vi "Write String.vi"(8 "error in (no error)":errorcluster, 11 "String":string) -> (0 "error out":errorcluster)   [LabVIEW 2015]
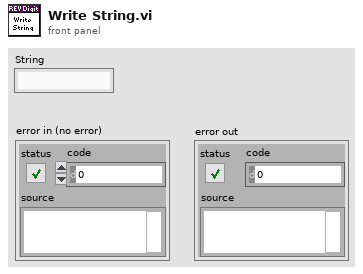
[diagram p1: front panel]
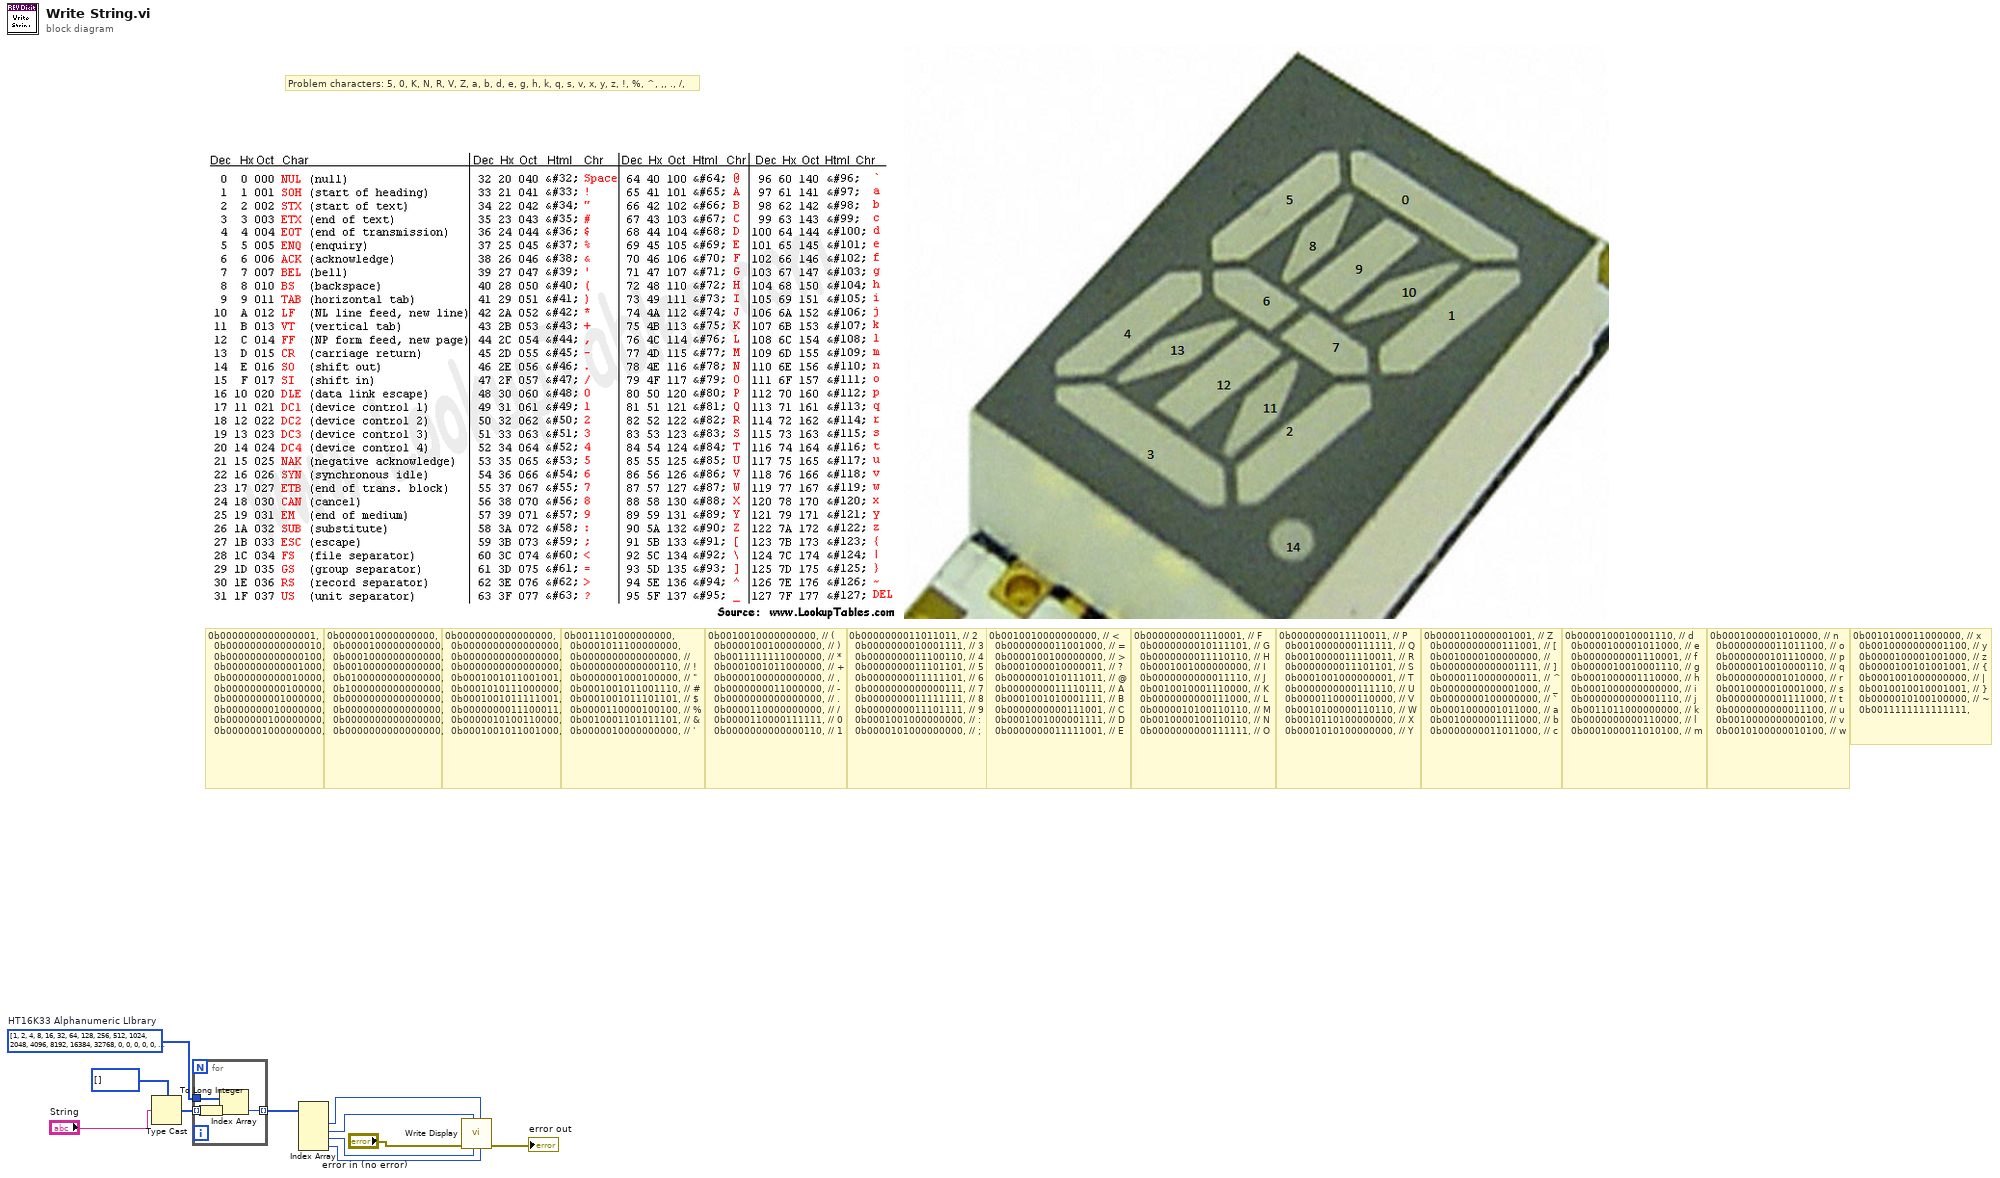
[diagram p0: block diagram]
diagram:
  w7 = u16[] [1, 2, 4, 8, 16, 32, 64, 128, 256, 512, 1024, 2048, 4096, 8192, 16384, 32768, 0, 0, 0, 0, 0, 0, 0, 0, 4809, 5568, 4857, 227, 1328, 4808, 14848, 5888, 0, 6, 544, 4814, 4845, 3108, 9053, 1024, 9216, 2304, 16320, 4800, 2048, 192, 0, 3072, 9279, 6, 219, 143, 230, 237, 253, 7, 255, 239, 4608, 2560, 9216, 200, 2304, 4227, 699, 247, 4751, 57, 4623, 249, 113, 189, 246, 4608, 30, 9328, 56, 1334, 8502, 63, 243, 8255, 8435, 237, 4609, 62, 3120, 10294, 11520, 5376, 3081, 57, 8448, 15, 3075, 8, 256, 4184, 8312, 216, 2190, 2136, 113, 1166, 4208, 4096, 14, 13824, 48, 4308, 4176, 220, 368, 1158, 80, 8328, 120, 28, 8196, 10260, 10432, 8204, 2120, 2377, 4608, 9353, 1312, 16383]  # HT16K33 Alphanumeric LIbrary
  # "Problem characters: 5, 0, K, N, R, V, Z, a, b, d, e, g, h, k, q, s, v, x, y, z, !, %, ^, ,, ., /,"
  # "0b0010100011000000, // x\n\t\t0b0010000000001100, // y\n\t\t0b0000100001001000, // z\n\t\t0b0000100101001001, // {\n\t\t0b0001001000000000, // |\n\t\t0b0010010010001001, // }\n\t\t0b0000010100100000, // ~\n\t\t0b0011111111111111,"
  # "0b0001000001010000, // n\n\t\t0b0000000011011100, // o\n\t\t0b0000000101110000, // p\n\t\t0b0000010010000110, // q\n\t\t0b0000000001010000, // r\n\t\t0b0010000010001000, // s\n\t\t0b0000000001111000, // t\n\t\t0b0000000000011100, // u\n\t\t0b0010000000000100, // v\n\t\t0b0010100000010100, // w"
  # "0b0000100010001110, // d\n\t\t0b0000100001011000, // e\n\t\t0b0000000001110001, // f\n\t\t0b0000010010001110, // g\n\t\t0b0001000001110000, // h\n\t\t0b0001000000000000, // i\n\t\t0b0000000000001110, // j\n\t\t0b0011011000000000, // k\n\t\t0b0000000000110000, // l\n\t\t0b0001000011010100, // m"
  # "0b0000000000000001,\n\t\t0b0000000000000010,\n\t\t0b0000000000000100,\n\t\t0b0000000000001000,\n\t\t0b0000000000010000,\n\t\t0b0000000000100000,\n\t\t0b0000000001000000,\n\t\t0b0000000010000000,\n\t\t0b0000000100000000,\n\t\t0b0000001000000000,"
  # "0b0000110000001001, // Z\n\t\t0b0000000000111001, // [\n\t\t0b0010000100000000, //\n\t\t0b0000000000001111, // ]\n\t\t0b0000110000000011, // ^\n\t\t0b0000000000001000, // _\n\t\t0b0000000100000000, // `\n\t\t0b0001000001011000, // a\n\t\t0b0010000001111000, // b\n\t\t0b0000000011011000, // c"
  # "0b0000000011110011, // P\n\t\t0b0010000000111111, // Q\n\t\t0b0010000011110011, // R\n\t\t0b0000000011101101, // S\n\t\t0b0001001000000001, // T\n\t\t0b0000000000111110, // U\n\t\t0b0000110000110000, // V\n\t\t0b0010100000110110, // W\n\t\t0b0010110100000000, // X\n\t\t0b0001010100000000, // Y"
  # "0b0000000001110001, // F\n\t\t0b0000000010111101, // G\n\t\t0b0000000011110110, // H\n\t\t0b0001001000000000, // I\n\t\t0b0000000000011110, // J\n\t\t0b0010010001110000, // K\n\t\t0b0000000000111000, // L\n\t\t0b0000010100110110, // M\n\t\t0b0010000100110110, // N\n\t\t0b0000000000111111, // O"
  # "0b0010010000000000, // <\n\t\t0b0000000011001000, // =\n\t\t0b0000100100000000, // >\n\t\t0b0001000010000011, // ?\n\t\t0b0000001010111011, // @\n\t\t0b0000000011110111, // A\n\t\t0b0001001010001111, // B\n\t\t0b0000000000111001, // C\n\t\t0b0001001000001111, // D\n\t\t0b0000000011111001, // E"
  # "0b0000000011011011, // 2\n\t\t0b0000000010001111, // 3\n\t\t0b0000000011100110, // 4\n\t\t0b0000000011101101, // 5\n\t\t0b0000000011111101, // 6\n\t\t0b0000000000000111, // 7\n\t\t0b0000000011111111, // 8\n\t\t0b0000000011101111, // 9\n\t\t0b0001001000000000, // :\n\t\t0b0000101000000000, // ;"
  # "0b0010010000000000, // (\n\t\t0b0000100100000000, // )\n\t\t0b0011111111000000, // *\n\t\t0b0001001011000000, // +\n\t\t0b0000100000000000, // ,\n\t\t0b0000000011000000, // -\n\t\t0b0000000000000000, // .\n\t\t0b0000110000000000, // /\n\t\t0b0000110000111111, // 0\n\t\t0b0000000000000110, // 1"
  # "0b0011101000000000,\n\t\t0b0001011100000000,\n\t\t0b0000000000000000, //\n\t\t0b0000000000000110, // !\n\t\t0b0000001000100000, // \"\n\t\t0b0001001011001110, // #\n\t\t0b0001001011101101, // $\n\t\t0b0000110000100100, // %\n\t\t0b0010001101011101, // &\n\t\t0b0000010000000000, // '"
  # "0b0000000000000000,\n\t\t0b0000000000000000,\n\t\t0b0000000000000000,\n\t\t0b0000000000000000,\n\t\t0b0001001011001001,\n\t\t0b0001010111000000,\n\t\t0b0001001011111001,\n\t\t0b0000000011100011,\n\t\t0b0000010100110000,\n\t\t0b0001001011001000,"
  # "0b0000010000000000,\n\t\t0b0000100000000000,\n\t\t0b0001000000000000,\n\t\t0b0010000000000000,\n\t\t0b0100000000000000,\n\t\t0b1000000000000000,\n\t\t0b0000000000000000,\n\t\t0b0000000000000000,\n\t\t0b0000000000000000,\n\t\t0b0000000000000000,"
  n1 = Type Cast(type=u8[] [], x="String") -> (*(type *) &x=w6:u8[])
  n2 = for {
    tunnel: w6 -> [w14] mode=indexing
    tunnel: w7 -> [w15]
    tunnel: [w13] -> w8 mode=indexing
    n3 = To Long Integer(number=w14) -> (32bit integer=w12:i32)
    n4 = Index Array(array=w15, index=w12) -> (element=w13:u16)
  }
  n5 = Index Array(array=w8) -> (element #1=w2:u16, element #2=w1:u16, element #3=w9:u16, element #4=w10:u16)  [unwired: 4 in]
  n6 = call "Write Display.vi"("D3"=w10, "D0"=w2, "D2"=w9, "D1"=w1, "error in (no error)"="error in (no error)") -> ("error out"=→"error out":errorcluster)  [unwired: 6 in]
